vi "Write Measurement Parameters.vi"(8 "error in (no error)":errorcluster, 10 "String Database.lvlibp:String Dictionary":refnum<class "String Database.lvclass">=refnum, 11 "Measurement Interface in":refnum<class "Measurement Interface.lvclass">=refnum) -> (0 "error out":errorcluster, 3 "Measurement Interface out":refnum<class "Measurement Interface.lvclass">)   [LabVIEW 2016, in "Measurement Interface.lvlib" / "Measurement Interface.lvclass"]
uses:
  Measurement Interface.lvclass
  Plugins/String Database.lvlibp/String Database.lvclass
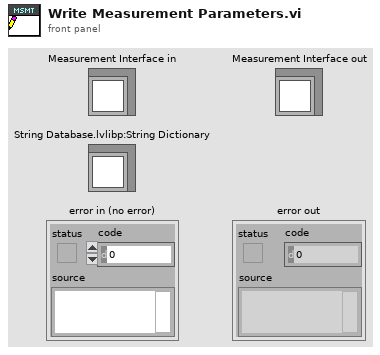
[diagram p1: front panel]
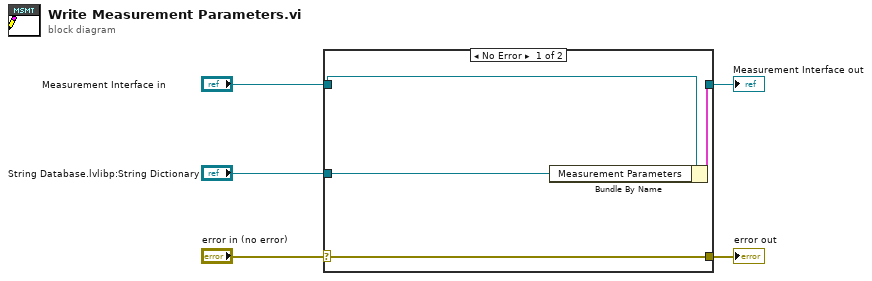
[diagram p0: block diagram]
diagram:
  n1 = case shown="No Error" "error in (no error)" {
    selector: "error in (no error)" -> [w9 w10]
    tunnel: [w9 w10] -> w4
    tunnel: [w7 w11] -> w2
    tunnel: "Measurement Interface in" -> [w8 w11]
    tunnel: "String Database.lvlibp:String Dictionary" -> [w6 _]
    frame No Error {
      n2 = Bundle By Name(cluster=w8, "Measurement Parameters"=w6) -> (w7:cluster{})
    }
    frame Error {
    }
  }
  "error out" <- w4
  "Measurement Interface out" <- w2
